vi "SetBEC.vi"(8 "error in (no error)":errorcluster, 10 "ecin100ns":u64=1, 11 "board_sel":u32=1) -> (0 "error out":errorcluster)   [LabVIEW 2015, in "ESLSCDLL.lvlib"]
uses:
  ESLSCDLL.lvlib
  ESLSCDLL.dll
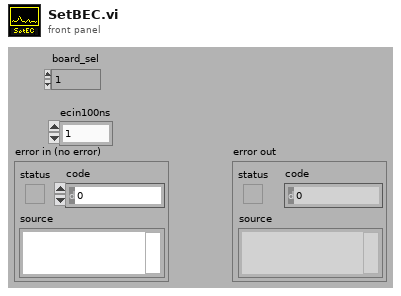
[diagram p1: front panel]
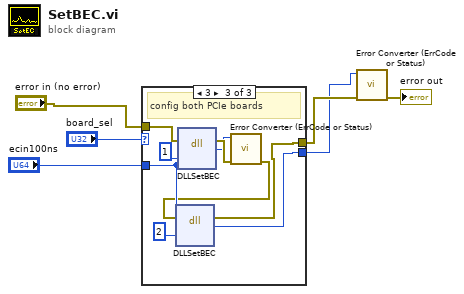
[diagram p0: block diagram]
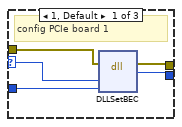
[diagram p2: hidden frame]
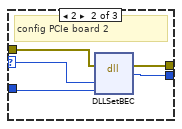
[diagram p3: hidden frame]
diagram:
  n1 = case shown="3" "board_sel" {
    selector: "board_sel" -> [w10 w15 _]
    tunnel: "ecin100ns" -> [w11 w16 w23]
    tunnel: "error in (no error)" -> [w9 w14 w22]
    tunnel: [w8 w13 w18] -> w3
    tunnel: [w7 w12 w17] -> w2
    frame 1, Default {
      # "config PCIe board 1"
      n2 = dll-call lib="C:/Users/flori/Nextcloud/Dokumente/Stresing/Windows/lv64/board.vis/ESLSCDLL.dll" fn="DLLSetBEC" ("lwlscdll.dll:DLLSetTemp")(error in=w9, "drv"=w10, "ecin100ns"=w11) -> (error out=w8:errorcluster, "es_status_codes"=w7:i32)  [unwired: 4 in, 1 out]
    }
    frame 2 {
      # "config PCIe board 2"
      n3 = dll-call lib="C:/Users/flori/Nextcloud/Dokumente/Stresing/Windows/lv64/board.vis/ESLSCDLL.dll" fn="DLLSetBEC" ("lwlscdll.dll:DLLSetTemp")(error in=w14, "drv"=w15, "ecin100ns"=w16) -> (error out=w13:errorcluster, "es_status_codes"=w12:i32)  [unwired: 4 in, 1 out]
    }
    frame 3 {
      # "config both PCIe boards"
      n4 = dll-call lib="C:/Users/flori/Nextcloud/Dokumente/Stresing/Windows/lv64/board.vis/ESLSCDLL.dll" fn="DLLSetBEC" ("lwlscdll.dll:DLLSetTemp")(error in=w22, "drv"=u32 1, "ecin100ns"=w23) -> (error out=w21:errorcluster, "es_status_codes"=w20:i32)  [unwired: 4 in, 1 out]
      n5 = call "Error Converter (ErrCode or Status).vi"("error in (no error)"=w21, "error code"=w20) -> ("error out"=w19:errorcluster)  [unwired: 9 in]
      n6 = dll-call lib="C:/Users/flori/Nextcloud/Dokumente/Stresing/Windows/lv64/board.vis/ESLSCDLL.dll" fn="DLLSetBEC" ("lwlscdll.dll:DLLSetTemp")(error in=w19, "drv"=u32 2, "ecin100ns"=w23) -> (error out=w18:errorcluster, "es_status_codes"=w17:i32)  [unwired: 4 in, 1 out]
    }
  }
  n7 = call "Error Converter (ErrCode or Status).vi"("error in (no error)"=w3, "error code"=w2) -> ("error out"=→"error out":errorcluster)  [unwired: 9 in]
